vi "Waveform_Read Write Name.vi"(7 "Read(f)\nWrite(t)":T1, 10 "Name":string, 11 "Raw Data Waveform":T2) -> (2 "Name Out":string, 3 "Raw Data Waveform Out":T2)   [LabVIEW 2020]
uses:
  Universal Controls/Waveform_Data.ctl
  Universal Controls/Read Write Button.ctl
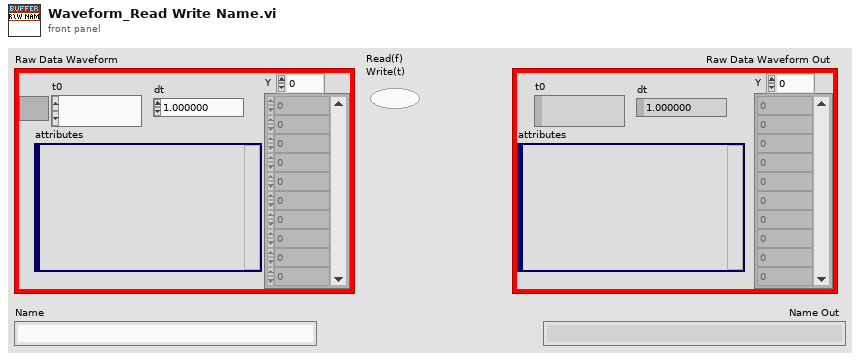
[diagram p1: front panel]
types:
  T1 = typedef "Read Write Button.ctl" = bool
  T2 = typedef "Waveform_Data.ctl" = waveform(dbl)
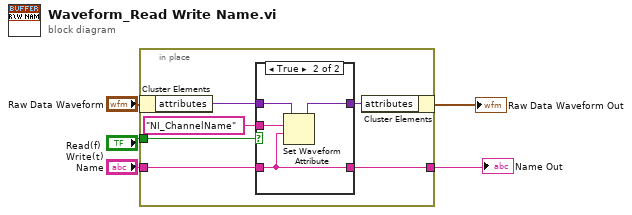
[diagram p0: block diagram]
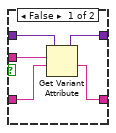
[diagram p2: hidden frame]
diagram:
  n1 = in-place {
    in-place-border: "Name" -> [w10]
    in-place-border: [w9] -> w1
    in-place-border: "Read(f)\nWrite(t)" -> [w6]
    n2 = in-place-cluster #1("Raw Data Waveform") -> ("attributes"=w8:variant)
    n3 = case shown="True" w6 {
      tunnel: "NI_ChannelName" ("name") -> [w14 w20]
      tunnel: w10 -> [w13 w18]
      tunnel: [w15 w19] -> w7
      tunnel: [w12 w18] -> w9
      tunnel: w8 -> [w16 w17]
      frame False {
        n4 = Get Variant Attribute(Variant=w16, name=w14, default value (empty Variant)=w13) -> (duplicate Variant=w15:variant, value=w12:string)  [unwired: 1 in, 2 out]
      }
      frame True {
        n5 = Set Waveform Attribute(5:w18, 6:w20, 7:w17) -> (3:w19:variant)  [unwired: 1 in, 2 out]
      }
    }
    n6 = in-place-cluster #1("attributes"=w7) -> (→"Raw Data Waveform Out":T2)
  }
  "Name Out" <- w1
